vi "TwChangePeakTable.vi"(0 "error in (no error)":errorcluster, 1 "filename":string, 2 "newPeakPar":string, 3 "nbrNewPeakPar":i32, 4 "compressionLevel":i32) -> (5 "error out":errorcluster)   [LabVIEW 2009]
uses:
  TwH5Dll.dll
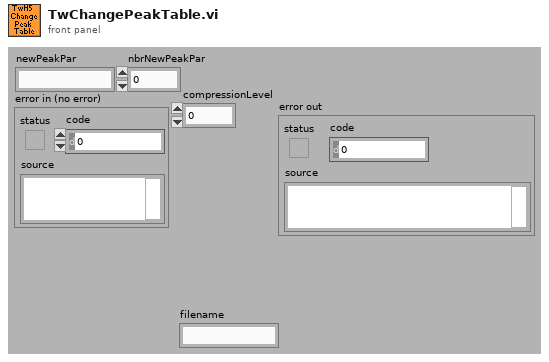
[diagram p1: front panel]
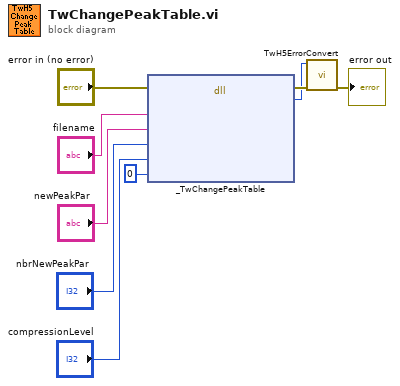
[diagram p0: block diagram]
diagram:
  n1 = dll-call lib="C:/src/85_TofDaq_current/DllWrappers/LabView/TwH5Dll/TwH5Dll.dll" fn="_TwChangePeakTable"(error in="error in (no error)", "filename"="filename", "newPeakPar"="newPeakPar", "nbrNewPeakPar"="nbrNewPeakPar", "compressionLevel"="compressionLevel", "callback"=u32 0) -> (error out=w8:errorcluster, "TwRetVal"=w7:i32)  [unwired: 7 in, 1 out]
  n2 = call "TwH5ErrorConvert.vi"("error in (no error)"=w8, "error code"=w7) -> ("error out"=→"error out":errorcluster)  [unwired: 9 out]
